vi "Is Interface Or LabVIEW Object Blue.vi"(8 "error in (no error)":errorcluster, 10 "Application:All VIs In Memory":string[](array[string]), 11 "LabVIEW Object":refnum<class>) -> (0 "error out":errorcluster, 3 "Is Class?":bool)   [LabVIEW 2020, in "BlueSerialization.lvlib" / "BlueSerializer.lvclass"]
uses:
  BlueSerializer.lvclass
  BlueSerializer.lvclass/BlueSerializer.ctl
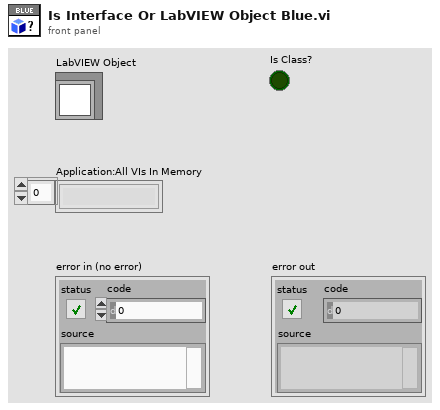
[diagram p1: front panel]
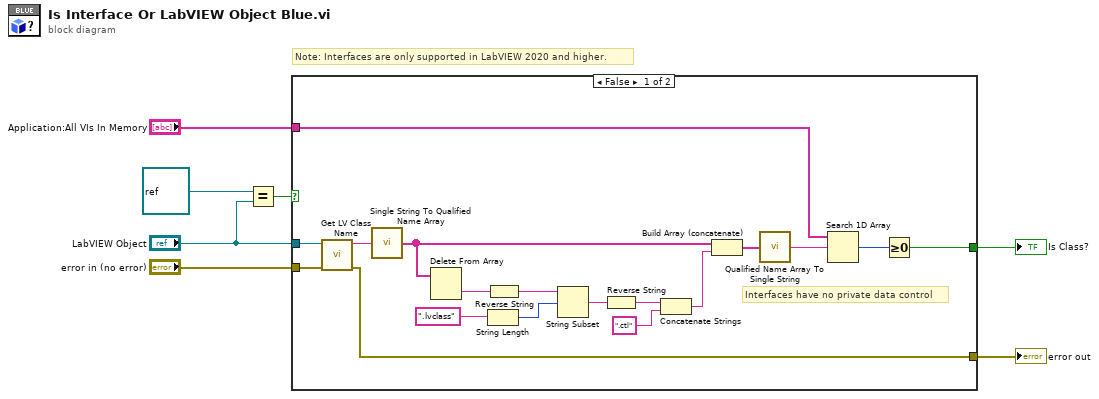
[diagram p0: block diagram]
diagram:
  # "Note: Interfaces are only supported in LabVIEW 2020 and higher."
  n1 = Equal?(x=refnum<class> refnum ("y"), y="LabVIEW Object") -> (x = y?=w6:bool)
  n2 = case shown="False" w6 {
    selector: w6 -> [_ w27]
    tunnel: "LabVIEW Object" -> [w25 _]
    tunnel: [w8 w27] -> w7
    tunnel: "error in (no error)" -> [w12 w26]
    tunnel: [w11 w26] -> w2
    tunnel: "Application:All VIs In Memory" -> [w10 _]
    frame False {
      # "Interfaces have no private data control"
      n3 = call <vilib>:"Get LV Class Name.vi"("error in (no error)"=w12, "object"=w25) -> ("error out"=w11:errorcluster, "class name"=w20:string)  [unwired: 8 in]
      n4 = call <vilib>:"Single String To Qualified Name Array.vi"("Fully Qualified String"=w20) -> ("Fully Qualified Array"=w19:string[])
      n5 = Delete From Array(array=w19) -> (deleted portion=w18:string)  [unwired: 2 in, 1 out]
      n6 = String Length(string=".lvclass") -> (length=w23:i32)
      n7 = Reverse String(1:w18) -> (0:w22:string)
      n8 = String Subset(string=w22, offset (0)=w23) -> (substring=w21:string)  [unwired: 1 in]
      n9 = Reverse String(1:w21) -> (0:w17:string)
      n10 = Concatenate Strings(w17, ".ctl" ("string")) -> (w15:string)
      n11 = Build Array (concatenate)(w19, w15) -> (w14:string[])
      n12 = call <vilib>:"Qualified Name Array To Single String.vi"("Fully Qualified Array"=w14) -> ("Fully Qualified String"=w13:string)
      n13 = Search 1D Array(1D array=w10, element=w13) -> (index of element=w9:i32)  [unwired: 1 in]
      n14 = Greater Or Equal To 0?(x=w9) -> (x >= 0?=w8:bool)
    }
    frame True {
    }
  }
  "Is Class?" <- w7
  "error out" <- w2
